vi "Image_Folder.vi"(8 "New":i32, 9 "Old":i32, 10 "Other":i32, 11 "input cluster":T1={"system"={"info"={"menuSelect"=0, "version"=0, "serial"="Test Sample", "captureActive"=FALSE, "captureBegin"=FALSE, "emptyAndRefill"=FALSE}, "userInfo"={"operatorName"="", "date"=timestamp(2713993200 s since 1904-01-01)}, "camera"={"exposureTime"=0, "aperture"=enum."Item 0", "framerate"=0, "framerateMax"=500, "legacyAttributes"=FALSE}}, "connections"={"arduino"={"connection"="MRJ", "status"=FALSE, "openState"=FALSE, "emptyStart"=0}, "pump"={"connection"="MRJ", "status"=FALSE, "command"="", "dispenseSpeed"=100, "flushSize"=100}, "camera"={"cam1"={"connection"="", "status"=FALSE}, "cam2"={"connection"="", "status"=FALSE}}}, "queue"={"process"={"cam1"=refnum, "cam2"=refnum, "queueSize"=0}, "save"={"cam1"=refnum, "cam2"=refnum, "queueSize"=0}, "overloadThreshold"=0}, "imageProcess"={"cam1"={"preAllocation"={"image"="Station", "originalDisplay"="Station", "originalRgb"="Station", "binary"="Station", "save"="Station", "calibrationFull"=refnum, "calibrationDetect"=refnum}, "calibration"={"pathFull"=path "C:/Users/au540322/Desktop/IHS_Project/images/Debris/Debris_0/Debris_0_2019_06_01-23-32-49-686.PNG", "pathDetect"=path "C:/Users/au540322/Desktop/IHS_Project/images/Debris/Debris_0/Debris_0_2019_06_01-23-32-49-686.PNG", "ROI"={"Left"=0, "Top"=0, "Right"=0, "Bottom"=0, "Rotation"=0.0}}}, "cam2"={"preAllocation"={"image"=refnum, "originalDisplay"=refnum, "originalRgb"=refnum, "binary"=refnum, "save"=refnum, "calibrationFull"=refnum, "calibrationDetect"=refnum}, "calibration"={"pathFull"=path "C:/Users/au540322/Desktop/IHS_Project/images/Debris/Debris_0/Debris_0_2019_06_01-23-32-49-686.PNG", "pathDetect"=path "C:/Users/au540322/Desktop/IHS_Project/images/Debris/Debris_0/Debris_0_2019_06_01-23-32-49-686.PNG", "ROI"={"Left"=0, "Top"=0, "Right"=0, "Bottom"=0, "Rotation"=0.0}}}, "process"={"planeExtract"=refnum, "planeSubtract"=refnum, "cropMask"=refnum}, "detection"={"sampleTimeout"=500, "sizeThreshold"=500, "detectionRegionPct"=0.0}}, "sampleData"={"sampleId"="", "projectId"="", "voucherID"="", "speciesName"="", "collectionDate"=timestamp(2713993200 s since 1904-01-01), "sampleStation"="", "location"="", "lat"=0.0, "lon"=0.0, "determiner"="", "sex"="", "otherNotes"=""}, "Session In"=""} {"sampleData"."collectionDate" format="%<%Y-%m-%d>T"; "imageProcess"."detection"."sizeThreshold" min=1; "imageProcess"."cam2"."calibration"."ROI"."Rotation" format="%.2f"; "imageProcess"."cam2"."calibration"."ROI"."Left" scale=0.0..1024.0; "imageProcess"."cam2"."calibration"."ROI"."Right" scale=0.0..1024.0; "imageProcess"."cam1"."calibration"."ROI"."Rotation" format="%.2f"; "imageProcess"."cam1"."calibration"."ROI"."Left" scale=0.0..1024.0; "imageProcess"."cam1"."calibration"."ROI"."Right" scale=0.0..1024.0; "queue"."overloadThreshold" min=1; "queue"."save"."queueSize" min=1; "queue"."process"."queueSize" min=1; "connections"."pump"."flushSize" min=1; "connections"."pump"."dispenseSpeed" min=1; "system"."camera"."framerateMax" min=1; "system"."userInfo"."date" format="%<%Y-%m-%dT%H:%M:%S+%z>T"; "system"."info"."version" items=["Standard", "XL"]; "system"."info"."menuSelect" items=["Session Data", "Extended Setup", "Buffer", "Camera", "Dispenser", "Stats", "Connections"]}) -> (2 "Subfolder Name":string, 3 "Subfolder Path":string)   [LabVIEW 2022 SP3]
uses:
  controls/Data.ctl
  <vilib>/userdefined/High Color/IMAQdx.ctl
  <vilib>/vision/Image Controls.llb/IMAQ Image.ctl
panel:
  out "error out 2":errorcluster
  out "error out":errorcluster
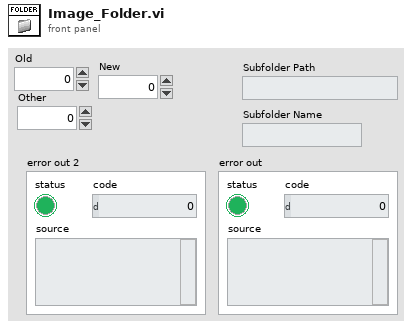
[diagram p1: front panel]
types:
  T1 = typedef "Data.ctl" = cluster{"system":cluster{"info":cluster{"menuSelect":u16, "version":u16, "serial":string, "captureActive":bool, "captureBegin":bool, "emptyAndRefill":bool}, "userInfo":cluster{"operatorName":string, "date":timestamp}, "camera":cluster{"exposureTime":i32, "aperture":enum32{"Item 0", "Item 1", "Item 2", "Item 3"}, "framerate":i32, "framerateMax":i32, "legacyAttributes":bool}}, "connections":cluster{"arduino":cluster{"connection":refnum<visa-resource-name>, "status":bool, "openState":bool, "emptyStart":u32}, "pump":cluster{"connection":refnum<visa-resource-name>, "status":bool, "command":string, "dispenseSpeed":i32, "flushSize":i32}, "camera":cluster{"cam1":cluster{"connection":T2, "status":bool}, "cam2":cluster{"connection":T2, "status":bool}}}, "queue":cluster{"process":cluster{"cam1":refnum<queue>, "cam2":refnum<queue>, "queueSize":i32}, "save":cluster{"cam1":refnum<queue>, "cam2":refnum<queue>, "queueSize":i32}, "overloadThreshold":i32}, "imageProcess":cluster{"cam1":cluster{"preAllocation":cluster{"image":T3, "originalDisplay":T3, "originalRgb":T3, "binary":T3, "save":T3, "calibrationFull":T3, "calibrationDetect":T3}, "calibration":cluster{"pathFull":path, "pathDetect":path, "ROI":T4}}, "cam2":cluster{"preAllocation":cluster{"image":T3, "originalDisplay":T3, "originalRgb":T3, "binary":T3, "save":T3, "calibrationFull":T3, "calibrationDetect":T3}, "calibration":cluster{"pathFull":path, "pathDetect":path, "ROI":T4}}, "process":cluster{"planeExtract":T3, "planeSubtract":T3, "cropMask":T3}, "detection":cluster{"sampleTimeout":i32, "sizeThreshold":i32, "detectionRegionPct":dbl}}, "sampleData":cluster{"sampleId":string, "projectId":string, "voucherID":string, "speciesName":string, "collectionDate":timestamp, "sampleStation":string, "location":string, "lat":dbl, "lon":dbl, "determiner":string, "sex":string, "otherNotes":string}, "Session In":T2}
  T2 = typedef "IMAQdx.ctl" = refnum<k21>
  T3 = typedef "IMAQ Image.ctl" = refnum<image>
  T4 = typedef "IMAQ Rectangle" = cluster{"Left":i32, "Top":i32, "Right":i32, "Bottom":i32, "Rotation":dbl}
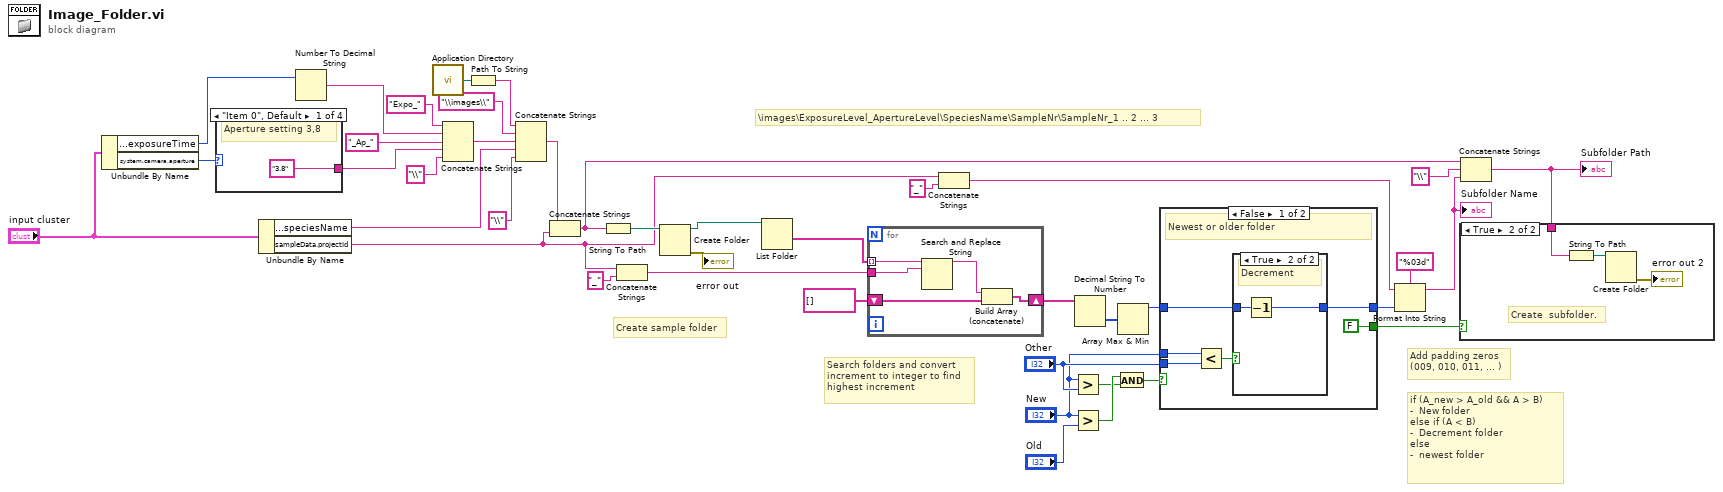
[diagram p0: block diagram]
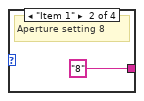
[diagram p2: hidden frame]
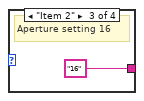
[diagram p3: hidden frame]
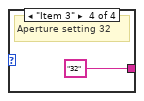
[diagram p4: hidden frame]
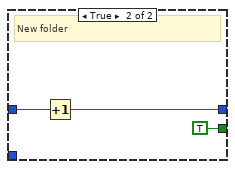
[diagram p6: hidden frame]
diagram:
  # "Add padding zeros\n(009, 010, 011, ... )"
  # "\\images\\ExposureLevel_ApertureLevel\\SpeciesName\\SampleNr\\SampleNr_1 .. 2 ... 3"
  # "if (A_new > A_old && A > B)\n-  New folder\nelse if (A < B)\n-  Decrement folder\nelse \n-  newest folder"
  # "Search folders and convert \nincrement to integer to find\nhighest increment"
  # "Create sample folder"
  n1 = Unbundle By Name("input cluster") -> ("system.camera.exposureTime"=w10:i32, "system.camera.aperture"=w7:enum32{"Item 0", "Item 1", "Item 2", "Item 3"})
  n2 = case shown="\"Item 0\", Default" w7 {
    tunnel: ["3.8" "8" "16" "32"] -> w4
    frame "Item 0", Default {
      # "Aperture setting 3,8"
    }
    frame "Item 1" {
      # "Aperture setting 8"
    }
    frame "Item 2" {
      # "Aperture setting 16"
    }
    frame "Item 3" {
      # "Aperture setting 32"
    }
  }
  n3 = Unbundle By Name("input cluster") -> ("sampleData.speciesName"=w15:string, "sampleData.projectId"=w13:string)
  n4 = Number To Decimal String(number=w10) -> (decimal integer string=w5:string)  [unwired: 1 in]
  n5 = call <vilib>:"Application Directory.vi"() -> ("Application Directory"=w34:path)
  n6 = Concatenate Strings("Expo_" ("string"), w5, "_Ap_" ("string"), w4, "\\" ("string")) -> (w2:string)
  n7 = Path To String(path=w34) -> (string=w35:string)
  n8 = Concatenate Strings(w35, "\\images\\" ("string"), w2, w15, "\\" ("string")) -> (w14:string)
  n9 = Concatenate Strings(w14, w13) -> (w12:string)
  n10 = String To Path(string=w12) -> (path=w37:path)
  n11 = Concatenate Strings(w13, "_" ("string")) -> (w32:string)
  n12 = Create Folder(path (use dialog)=w37) -> (created path=w40:path, error out=→"error out":errorcluster)  [unwired: 2 in, 1 out]
  n13 = List Folder(path=w40) -> (folder names=w33:string[])  [unwired: 3 in, 3 out]
  n14 = for {
    tunnel: w33 -> [w50] mode=indexing
    tunnel: w32 -> [w49]
    shift-right: [w47] -> w30
    shift-left: string[] [] -> [w46]
    n15 = Search and Replace String(input string=w50, search string=w49) -> (result string=w48:string)  [unwired: 6 in, 3 out]
    n16 = Build Array (concatenate)(w48, w46) -> (w47:string[])
  }
  n17 = Concatenate Strings(w13, "_" ("string")) -> (w26:string)
  n18 = Greater?(x="New", y="Other") -> (0:w23:bool)
  n19 = Greater?(x="New", y="Old") -> (0:w24:bool)
  n20 = Decimal String To Number(string=w30) -> (number=w29:i32[])  [unwired: 2 in, 1 out]
  n21 = And(x=w24, y=w23) -> (x .and. y?=w22:bool)
  n22 = Array Max & Min(array=w29) -> (max value=w18:i32)  [unwired: 3 out]
  n23 = case shown="False" w22 {
    tunnel: "Other" -> [w56 _]
    tunnel: "New" -> [w55 _]
    tunnel: [FALSE ("New sample (F)") TRUE ("New sample (F)")] -> w19
    tunnel: w18 -> [w53 w61]
    tunnel: [w52 w60] -> w17
    frame False {
      # "Newest or older folder"
      n24 = Less?(x=w55, y=w56) -> (x < y?=w54:bool)
      n25 = case shown="True" w54 {
        tunnel: w53 -> [w57 w59]
        tunnel: [w57 w58] -> w52
        frame False {
          # "Newest folder"
        }
        frame True {
          # "Decrement"
          n26 = Decrement(x=w59) -> (x-1=w58:i32)
        }
      }
    }
    frame True {
      # "New folder"
      n27 = Increment(x=w61) -> (x+1=w60:i32)
    }
  }
  n28 = Format Into String(format string="%03d", initial string=w26, w17) -> (resulting string=w27:string)  [unwired: 1 in, 1 out]
  "Subfolder Name" <- w27
  n29 = Concatenate Strings(w12, "\\" ("string"), w27) -> (w16:string)
  "Subfolder Path" <- w16
  n30 = case shown="True" w19 {
    tunnel: w16 -> [_ w63]
    frame False {
    }
    frame True {
      # "Create  subfolder."
      n31 = String To Path(string=w63) -> (path=w64:path)
      n32 = Create Folder(path (use dialog)=w64) -> (error out=→"error out 2":errorcluster)  [unwired: 2 in, 2 out]
    }
  }
